vi "Test color map.vi"() -> ()   [LabVIEW 2015]
uses:
  Type Defs/Color Map.ctl
panel:
  in  "Color Map":T1=enum."Green"
  out "Intensity Graph":dbl[][](graph)=[[0.0, 0.0], [1.0, 1.0], [2.0, 2.0], [3.0, 3.0], [4.0, 4.0], [5.0, 5.0], [6.0, 6.0], [7.0, 7.0], [8.0, 8.0], [9.0, 9.0], [10.0, 10.0], [11.0, 11.0], [12.0, 12.0], [13.0, 13.0], [14.0, 14.0], [15.0, 15.0], [16.0, 16.0], [17.0, 17.0], [18.0, 18.0], [19.0, 19.0], [20.0, 20.0], [21.0, 21.0], [22.0, 22.0], [23.0, 23.0], [24.0, 24.0], [25.0, 25.0], [26.0, 26.0], [27.0, 27.0], [28.0, 28.0], [29.0, 29.0], [30.0, 30.0], [31.0, 31.0], [32.0, 32.0], [33.0, 33.0], [34.0, 34.0], [35.0, 35.0], [36.0, 36.0], [37.0, 37.0], [38.0, 38.0], [39.0, 39.0], [40.0, 40.0], [41.0, 41.0], [42.0, 42.0], [43.0, 43.0], [44.0, 44.0], [45.0, 45.0], [46.0, 46.0], [47.0, 47.0], [48.0, 48.0], [49.0, 49.0], [50.0, 50.0], [51.0, 51.0], [52.0, 52.0], [53.0, 53.0], [54.0, 54.0], [55.0, 55.0], [56.0, 56.0], [57.0, 57.0], [58.0, 58.0], [59.0, 59.0], [60.0, 60.0], [61.0, 61.0], [62.0, 62.0], [63.0, 63.0], [64.0, 64.0], [65.0, 65.0], [66.0, 66.0], [67.0, 67.0], [68.0, 68.0], [69.0, 69.0], [70.0, 70.0], [71.0, 71.0], [72.0, 72.0], [73.0, 73.0], [74.0, 74.0], [75.0, 75.0], [76.0, 76.0], [77.0, 77.0], [78.0, 78.0], [79.0, 79.0], [80.0, 80.0], [81.0, 81.0], [82.0, 82.0], [83.0, 83.0], [84.0, 84.0], [85.0, 85.0], [86.0, 86.0], [87.0, 87.0], [88.0, 88.0], [89.0, 89.0], [90.0, 90.0], [91.0, 91.0], [92.0, 92.0], [93.0, 93.0], [94.0, 94.0], [95.0, 95.0], [96.0, 96.0], [97.0, 97.0], [98.0, 98.0], [99.0, 99.0]]
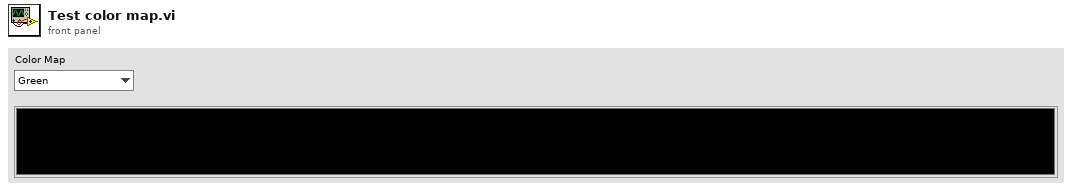
[diagram p1: front panel]
types:
  T1 = typedef "Color Map.ctl" = enum16{"Boring", "Fire", "Crazy", "Asylum", "Cubehelix", "Red", "Green", "Blue"}
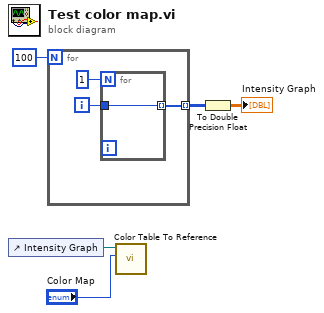
[diagram p0: block diagram]
diagram:
  n1 = control-ref of="Intensity Graph"() -> (w2:refnum<vi>)
  n2 = for {
    N: 100 -> [_]
    tunnel: [w7] -> w3 mode=indexing
    i -> [w8]
    n3 = for {
      N: 1 -> [_]
      tunnel: w8 -> [w9]
      tunnel: [w9] -> w7 mode=indexing
    }
  }
  n4 = call "Color Table To Reference.vi"("Color Map"="Color Map", "Intensity Graph Reference"=w2) -> ()  [unwired: 10 in]
  n5 = To Double Precision Float(number=w3) -> (double precision float=→"Intensity Graph":dbl[][])
